vi "MAIN_merFISH_move_to_ROI.vi"(0 "Data cluster":T3, 1 "queue piezo":refnum<queue>, 2 "queue ASI stage":refnum<queue>, 5 "merFISH mode":u16(ring) items=["Embryo", "Single ROI"], 7 "ROI manager Refnum":refnum<vi>, 9 "variant":variant, 11 "error in":errorcluster, 12 "XY positions Refnum":refnum<vi>, 13 "Global parameters IN":T1 {"# repetitions" min=0; "Dt (s)" min=0 step=1; "Filter list" items=["ET665lp", "zet405/488/561/640m", "None", "None", "None", "None"]}) -> (6 "XY positions OUT":dbl[][](array[numeric]), 8 "Next task":T2, 10 "XY graph":cluster{dbl[], dbl[]}[](array[cluster]), 14 "Global parameters out":T1 {"# repetitions" min=0; "Dt (s)" min=0 step=1; "Filter list" items=["ET665lp", "zet405/488/561/640m", "None", "None", "None", "None"]}, 15 "error out":errorcluster)   [LabVIEW 2015]
uses:
  CONTROLS/Q_ASI_stage_element.ctl
  CONTROLS/Q_MCL_piezo_element.ctl
  CONTROLS/Global parameters.ctl
  CONTROLS/Q_main_element.ctl
  GLOBAL/Global_MCL_piezo.vi
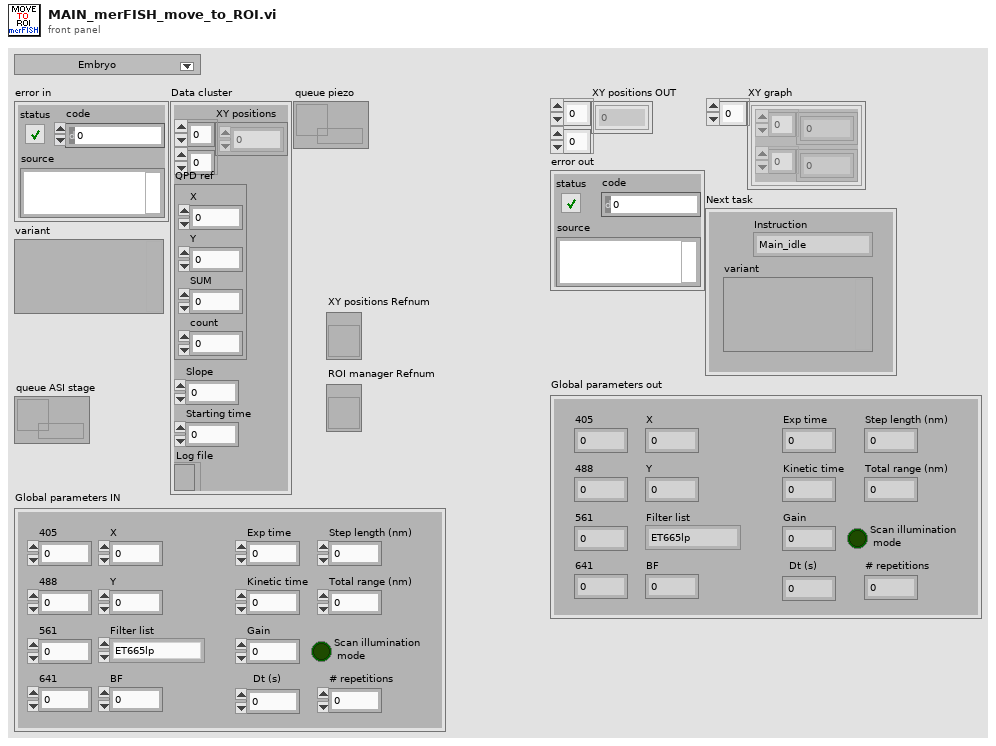
[diagram p1: front panel]
types:
  T1 = typedef "Global parameters.ctl" = cluster{"405":dbl, "488":dbl, "561":dbl, "641":dbl, "BF":dbl, "X":dbl, "Y":dbl, "Filter list":u16, "Exp time":sgl, "Kinetic time":sgl, "Gain":i32, "Step length (nm)":u32, "Total range (nm)":u32, "Scan illumination\n mode":bool, "Dt (s)":i32, "# repetitions":i32}
  T2 = typedef "Q_main_element.ctl" = cluster{"variant":variant, "Instruction":enum16{"Main_idle", "Main_initialize", "Main_initialize_TDMS", "Main_initialize_Queue", "Main_error", "Main_DAQ_initialization_results", "Main_ASI_initialization_results", "Main_Piezo_initialization_results", "Main_Valve_initialization_results", "Main_Pump_initialization_results", "Main_CAMERA_initialization_results", "Main_FPGA_initialization_results", "Main_DAQ_error", "Main_ASI_error", "Main_Piezo_error", "Main_CAMERA_error", "Main_Valve_error", "Main_Pump_error", "Main_FPGA_error", "Main_start_acquiring", "Main_not_acquiring", "Main_acquiring", "Main_stop_acquiring", "Main_change_exposure", "Main_change_z_scan_parameters", "Main_define_ROI", "Main_define_mosaic", "Main_read_kinetic_time", "Main_cooler", "Main_read_temperature", "Main_save_XY", "Main_load_XY", "Main_discard_XY", "Main_move_to_XY", "Main_measure_QPD", "Main_autofocus_calibration", "Main_autofocus_initialization", "Main_autofocus_stop", "Main_save_PID", "Main_change_H_valve_position", "Main_two_way_valve", "Main_save_movie", "Main_init_single_scan", "Main_single_scan", "Main_stop_single_scan", "Main_merFISH_illumination_parameters", "Main_merFISH_buffer_probe_list", "Main_merFISH_injections_procedure", "Main_merFISH_save_setpoint", "Main_merFISH_DAPI_parameters", "Main_merFISH_Brightfield_parameters", "Main_merFISH_save_embryo_ROI", "Main_merFISH_init", "Main_merFISH_resume", "Main_merFISH_start_autofocus", "Main_merFISH_open_close_valve_merFISH", "Main_merFISH_open_close_valve_photobleaching", "Main_merFISH_hybridization", "Main_merFISH_move_to_ROI", "Main_merFISH_wait_stabilization", "Main_merFISH_move_to_REF", "Main_merFISH_scan", "Main_merFISH_photobleaching_injection", "Main_merFISH_photobleaching", "Main_merFISH_send_email", "Main_merFISH_close", "Main_STOP"}}
  T3 = cluster{"XY positions":dbl[][], "Slope":dbl, "Starting time":dbl, "Log file":refnum<file>, "QPD ref":cluster{"X":sgl, "Y":sgl, "SUM":sgl, "count":u32}}
  T4 = cluster{"X":sgl, "Y":sgl, "SUM":sgl, "count":u32}
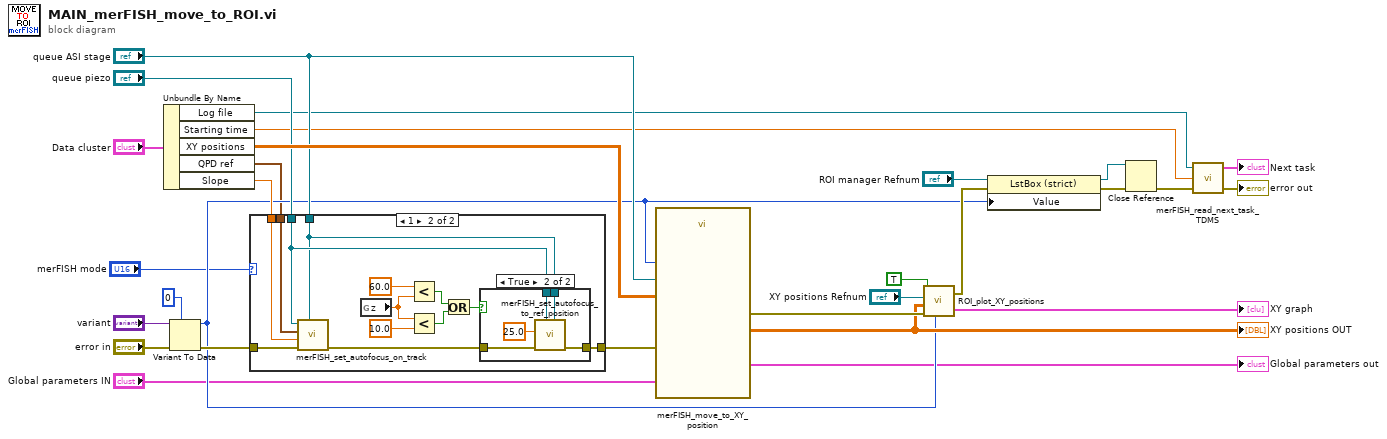
[diagram p0: block diagram]
diagram:
  n1 = Unbundle By Name("Data cluster") -> ("Log file"=w16:refnum<file>, "Starting time"=w15:dbl, "XY positions"=w20:dbl[][], "QPD ref"=w2:T4, "Slope"=w21:dbl)
  n2 = Variant To Data(error in="error in", type=0 ("ROI #"), Variant="variant") -> (data=w9:i32, error out=w27:errorcluster)
  n3 = case shown="1" "merFISH mode" {
    tunnel: [w30 w37] -> w29
    tunnel: w27 -> [w30 w35]
    tunnel: w21 -> [_ w34]
    tunnel: "queue piezo" -> [_ w33]
    tunnel: "queue ASI stage" -> [_ w32]
    tunnel: w2 -> [_ w31]
    frame 0, Default {
    }
    frame 1 {
      n4 = call "merFISH_set_autofocus_on_track.vi"("queue ASI stage"=w32, "error in"=w35, "Slope"=w34, "QPD ref"=w31, "queue piezo"=w33) -> ("error out"=w36:errorcluster)  [unwired: 4 in]
      n5 = global read "Global_MCL_piezo.vi" "z"() -> (w39:dbl)
      n6 = Less?(x=60.0, y=w39) -> (x < y?=w41:bool)
      n7 = Less?(x=w39, y=10.0) -> (x < y?=w42:bool)
      n8 = Or(x=w41, y=w42) -> (x .or. y?=w43:bool)
      n9 = case shown="True" w43 {
        tunnel: w36 -> [w44 w48]
        tunnel: [w44 w47] -> w37
        tunnel: w33 -> [_ w46]
        tunnel: w32 -> [_ w45]
        frame False {
        }
        frame True {
          n10 = call "merFISH_set_autofocus_to_ref_position.vi"("queue ASI stage"=w45, "queue piezo"=w46, "error in"=w48, "Ref"=25.0) -> ("error out"=w47:errorcluster)  [unwired: 7 in]
        }
      }
    }
  }
  n11 = call "merFISH_move_to_XY_position.vi"("ROI #"=w9, "Global parameters"="Global parameters IN", "queue ASI stage"="queue ASI stage", "error in"=w29, "XY positions"=w20) -> ("Global parameters out"=→"Global parameters out":T1, "error out"=w28:errorcluster, "XY positions"=w26:dbl[][])  [unwired: 4 in]
  "XY positions OUT" <- w26
  n12 = call "ROI_plot_XY_positions.vi"("Display?"=TRUE, "XYGraph Refnum"="XY positions Refnum", "XY positions"=w26, "error in"=w28, "ROI manager"=w9) -> ("error out"=w14:errorcluster, "XY graph"=→"XY graph":cluster{dbl[], dbl[]}[])
  n13 = property class="LstBox (strict)"(reference="ROI manager Refnum", error in=w14, "Value"=w9) -> (reference out=w11:refnum<vi>, error out=w12:errorcluster)
  n14 = Close Reference(reference=w11, error in (no error)=w12) -> (error out=w10:errorcluster)
  n15 = call "merFISH_read_next_task_TDMS.vi"("error in"=w10, "Starting time"=w15, "Log file"=w16) -> ("error out"=→"error out":errorcluster, "task"=→"Next task":T2)  [unwired: 1 in]
